vi "Fit RSS, AIC & BIC.vi"(6 "NL Fit Method":T1, 8 "Error In":errorcluster, 9 "DOF":i32, 10 "Best Fit":dbl[](array[numeric]), 11 "Data":dbl[](array[numeric])) -> (0 "Error Out":errorcluster, 1 "BIC":dbl, 2 "AIC":dbl, 3 "RSS":dbl)   [LabVIEW 2021, in "Fits.lvlib"]
uses:
  Fits.lvlib
  Nonlinear Fit Method.ctl
  <vilib>/Utility/error.llb/Error Cluster From Error Code.vi
  <vilib>/ErrorRing/Error Ring.xnode
panel:
  # "see the AlliGator License on the block diagram (Ctrl+E or Window:Show Block Diagram)"
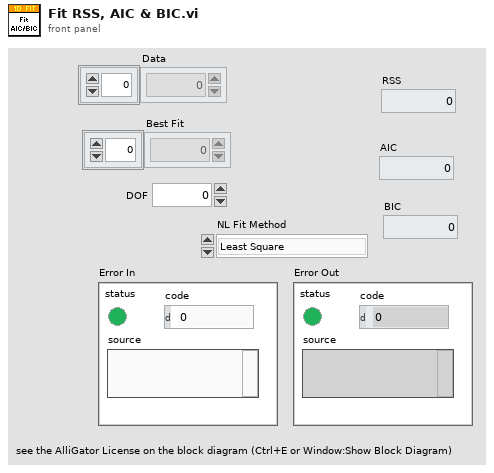
[diagram p1: front panel]
types:
  T1 = typedef "Fits.lvlib/Nonlinear Fit Method.ctl" = enum16{"Least Square", "Least Absolute Residual", "Bisquare", "MLE"}
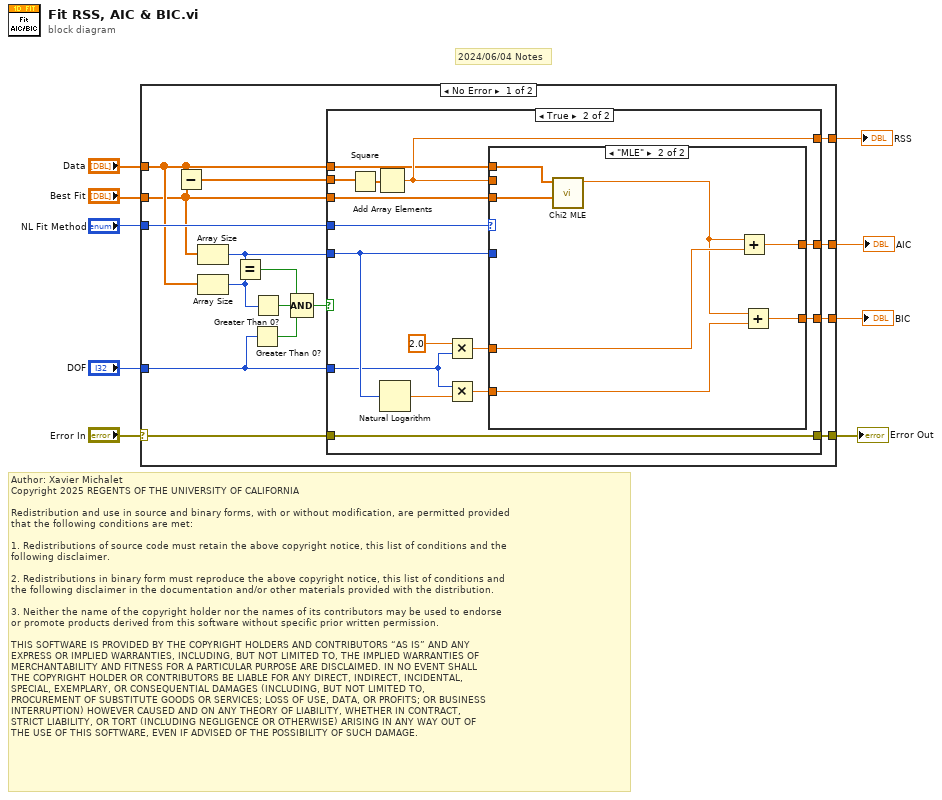
[diagram p0: block diagram]
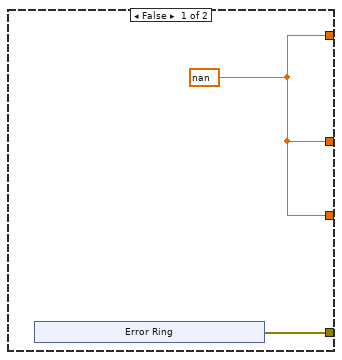
[diagram p2: hidden frame]
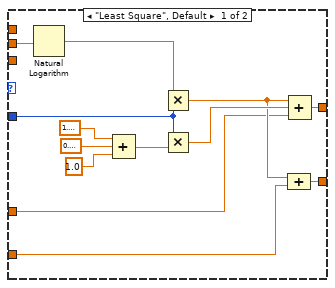
[diagram p3: hidden frame]
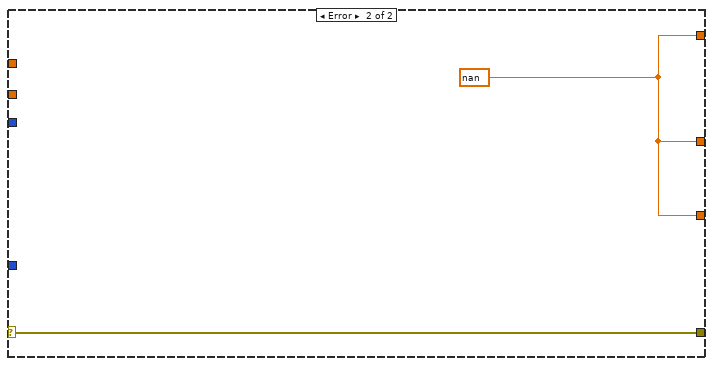
[diagram p4: hidden frame]
diagram:
  # "Author: Xavier Michalet\nCopyright 2025 REGENTS OF THE UNIVERSITY OF CALIFORNIA\n\nRedistribution and use in source and binary forms, with or without modification, are permitted provided\nthat the following conditions are met:\n\n1. Redistributions of source code must retain the above copyright notice, this list of conditions and the\nfollowing disclaimer.\n\n2. Redistributions in binary form must reproduce the above copyright notice, this list of conditions and\nthe following disclaimer in the documentation and/or other materials provided with the distribution.\n\n3. Neither the name of the copyright holder nor the names of its contributors may be used to endorse \nor promote products derived from this software without specific prior written permission.\n\nTHIS SOFTWARE IS PROVIDED BY THE COPYRIGHT HOLDERS AND CONTRIBUTORS “AS IS” AND ANY \nEXPRESS OR IMPLIED WARRANTIES, INCLUDING, BUT NOT LIMITED TO, THE IMPLIED WARRANTIES OF\nMERCHANTABILITY AND FITNESS FOR A PARTICULAR PURPOSE ARE DISCLAIMED. IN NO EVENT SHALL\nTHE COPYRIGHT HOLDER OR CONTRIBUTORS BE LIABLE FOR ANY DIRECT, INDIRECT, INCIDENTAL, \nSPECIAL, EXEMPLARY, OR CONSEQUENTIAL DAMAGES (INCLUDING, BUT NOT LIMITED TO, \nPROCUREMENT OF SUBSTITUTE GOODS OR SERVICES; LOSS OF USE, DATA, OR PROFITS; OR BUSINESS\nINTERRUPTION) HOWEVER CAUSED AND ON ANY THEORY OF LIABILITY, WHETHER IN CONTRACT, \nSTRICT LIABILITY, OR TORT (INCLUDING NEGLIGENCE OR OTHERWISE) ARISING IN ANY WAY OUT OF\nTHE USE OF THIS SOFTWARE, EVEN IF ADVISED OF THE POSSIBILITY OF SUCH DAMAGE."
  # "2024/06/04 Notes"
  n1 = case shown="No Error" "Error In" {
    selector: "Error In" -> [w13 w67]
    tunnel: "Data" -> [w11 _]
    tunnel: "Best Fit" -> [w10 _]
    tunnel: [w24 w68] -> w7
    tunnel: [w23 w68] -> w6
    tunnel: "DOF" -> [w19 _]
    tunnel: [w22 w68] -> w4
    tunnel: [w14 w67] -> w2
    tunnel: "NL Fit Method" -> [w12 _]
    frame No Error {
      n2 = Subtract(x=w11, y=w10) -> (x-y=w25:dbl[])
      n3 = Array Size(array=w10) -> (size(s)=w21:i32)
      n4 = Array Size(array=w11) -> (size(s)=w20:i32)
      n5 = Equal?(x=w21, y=w20) -> (x = y?=w17:bool)
      n6 = Greater Than 0?(x=w19) -> (x > 0?=w16:bool)
      n7 = Greater Than 0?(x=w20) -> (x > 0?=w18:bool)
      n8 = Compound Arithmetic op=AND(w17, w18, w16) -> (w15:bool)
      n9 = case shown="True" w15 {
        tunnel: w25 -> [_ w46]
        tunnel: [w27 w45] -> w24
        tunnel: [w27 w44] -> w23
        tunnel: [w27 w43] -> w22
        tunnel: w21 -> [_ w42]
        tunnel: w19 -> [_ w35]
        tunnel: [w26 w41] -> w14
        tunnel: w13 -> [_ w41]
        tunnel: w12 -> [_ w39]
        tunnel: w11 -> [_ w38]
        tunnel: w10 -> [_ w37]
        frame False {
          w27 = nan
          n10 = xnode "Error Ring"() -> ("error out"=w26:errorcluster)
        }
        frame True {
          n11 = Square(x=w46) -> (x^2=w40:dbl[])
          n12 = Add Array Elements(numeric array=w40) -> (sum=w45:dbl)
          n13 = Natural Logarithm(1:w42) -> (0:w36:dbl)
          n14 = Multiply(x=2.0, y=w35) -> (x*y=w32:dbl)
          n15 = Multiply(x=w35, y=w36) -> (x*y=w33:dbl)
          n16 = case shown="\"MLE\"" w39 {
            tunnel: w45 -> [w59 _]
            tunnel: [w58 w63] -> w44
            tunnel: [w57 w60] -> w43
            tunnel: w42 -> [w56 _]
            tunnel: w38 -> [_ w66]
            tunnel: w37 -> [_ w65]
            tunnel: w33 -> [w48 w61]
            tunnel: w32 -> [w47 w64]
            frame "Least Square", Default {
              n17 = Natural Logarithm(1:w59) -> (0:w55:dbl)
              n18 = Compound Arithmetic op=unknown(1.1447298858494002, 0.6931471805599453, 1.0 ("value")) -> (w51:dbl)
              n19 = Multiply(x=w55, y=w56) -> (x*y=w49:dbl)
              n20 = Multiply(x=w56, y=w51) -> (x*y=w50:dbl)
              n21 = Compound Arithmetic op=ADD(w49, w48) -> (w57:dbl)
              n22 = Compound Arithmetic op=ADD(w49, w50, w47) -> (w58:dbl)
            }
            frame "MLE" {
              n23 = call "Chi2 MLE.vi"("f(X)"=w65, "Y"=w66) -> ("chi2_mle"=w62:dbl)  [unwired: 9 in]
              n24 = Add(x=w62, y=w64) -> (x+y=w63:dbl)
              n25 = Add(x=w62, y=w61) -> (x+y=w60:dbl)
            }
          }
        }
      }
    }
    frame Error {
      w68 = nan
    }
  }
  "RSS" <- w7
  "AIC" <- w6
  "BIC" <- w4
  "Error Out" <- w2
